vi "SE5082_Output_OFF.vi"(8 "error in":errorcluster, 11 "VISA resource name in":refnum<visa-resource-name>="USB0::0x168C::0x5082::0000217419::INSTR") -> (0 "error out":errorcluster, 3 "VISA resource name out":refnum<visa-resource-name>="USB0::0x168C::0x5082::0000217419::INSTR")   [LabVIEW 2017]
panel:
  in  "Readout status?":bool
  in  "Read-out commands":string[](array[string])=[":INST 1;:VOLT?", ":INST 1;:VOLT:OFFS?", ":INST 1;:OUTP?", ":INST 2;:VOLT?", ":INST 2;:VOLT:OFFS?", ":INST 2;:OUTP?"]
  out "Input waveform commands":string[](array[string])=[":INST 1;:OUTP ON", ":INST 2;:OUTP ON"]
  out "Status output":string[](array[string])=["1.000e+00\n", "0.000e+00\n", "ON\n", "5.000e-01\n", "0.000e+00\n", "ON\n"]
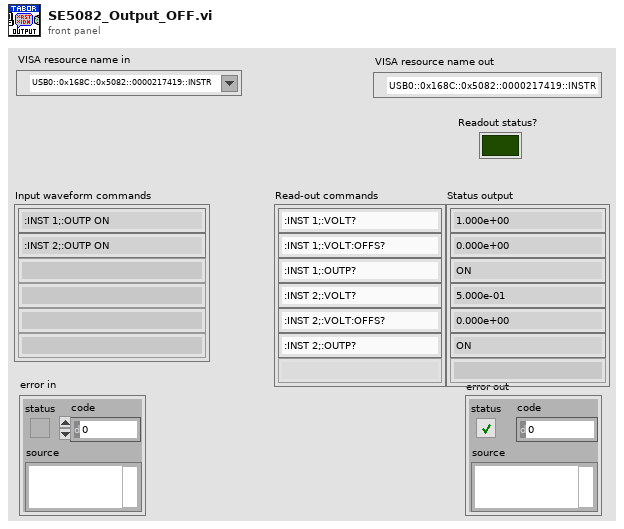
[diagram p1: front panel]
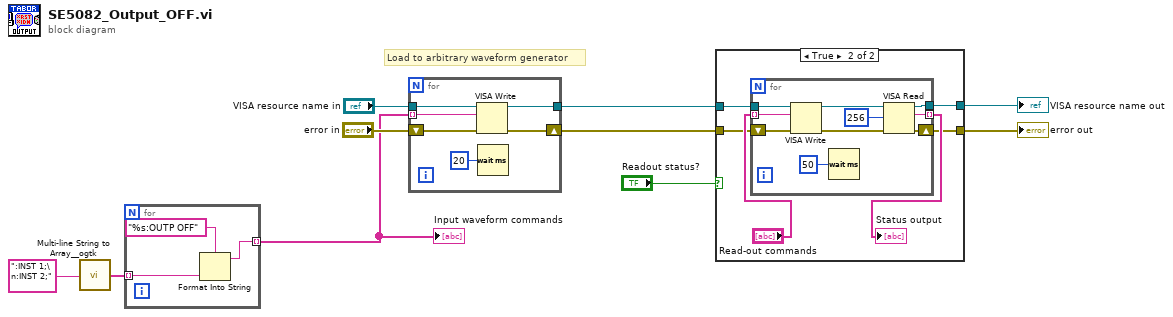
[diagram p0: block diagram]
diagram:
  # "Load to arbitrary waveform generator"
  n1 = call <userlib>:"Multi-line String to Array__ogtk.vi"("string"=":INST 1;\n:INST 2;" ("initial string")) -> ("lines"=w2:string[])
  n2 = for {
    tunnel: w2 -> [w11] mode=indexing
    tunnel: [w12] -> w1 mode=indexing
    n3 = Format Into String(format string="%s:OUTP OFF", w11) -> (resulting string=w12:string)  [unwired: 2 in, 1 out]
  }
  "Input waveform commands" <- w1
  n4 = for {
    tunnel: "VISA resource name in" -> [w19]
    tunnel: w1 -> [w18] mode=indexing
    shift-right: [w16] -> w7
    shift-left: "error in" -> [w17]
    tunnel: [w15] -> w8
    n5 = VISA Write(VISA resource name=w19, write buffer=w18, error in (no error)=w17) -> (VISA resource name out=w15:refnum<visa-resource-name>, error out=w16:errorcluster)  [unwired: 1 out]
    n6 = Wait (ms)(milliseconds to wait=u32 20) -> ()  [unwired: 1 out]
  }
  n7 = case shown="True" "Readout status?" {
    tunnel: w8 -> [w21 w25]
    tunnel: w7 -> [w20 w24]
    tunnel: [w20 w23] -> w6
    tunnel: [w21 w22] -> w5
    frame False {
    }
    frame True {
      n8 = for {
        tunnel: [w34] -> w27 mode=indexing
        shift-right: [w33] -> w23
        shift-left: w24 -> [w30]
        tunnel: w25 -> [w32]
        tunnel: "Read-out commands" -> [w31] mode=indexing
        tunnel: [w28] -> w22
        n9 = VISA Write(VISA resource name=w32, write buffer=w31, error in (no error)=w30) -> (VISA resource name out=w36:refnum<visa-resource-name>, error out=w35:errorcluster)  [unwired: 1 out]
        n10 = Wait (ms)(milliseconds to wait=u32 50) -> ()  [unwired: 1 out]
        n11 = VISA Read(VISA resource name=w36, byte count=u32 256, error in (no error)=w35) -> (VISA resource name out=w28:refnum<visa-resource-name>, read buffer=w34:string, error out=w33:errorcluster)  [unwired: 1 out]
      }
      "Status output" <- w27
    }
  }
  "error out" <- w6
  "VISA resource name out" <- w5
